vi "Get Configuration Version.vi"(8 "error in":errorcluster, 11 "data sharing framework custom device in":T1 format="%.0x") -> (0 "error out":errorcluster, 1 "version string":string, 2 "version":cluster{"major":u32, "minor":u32, "update":u32}, 3 "data sharing framework custom device out":T1 format="%.0x")   [LabVIEW 2020, in "Data Sharing Framework Custom Device Scripting.lvlib"]
doc: "Reads the version of the Data Sharing Framework custom device."
uses:
  Data Sharing Framework Custom Device Scripting.lvlib
  <vilib>/NI VeriStand/Custom Device API/Custom Device Item Ref.ctl
  DSF Shared.lvlib
  DSF System Explorer.lvlib
  <vilib>/NI VeriStand/Custom Device API/Custom Device API.lvlib
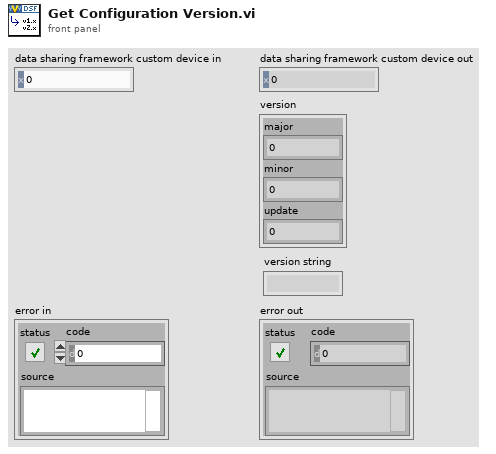
[diagram p1: front panel]
types:
  T1 = typedef "Custom Device API.lvlib/Custom Device Item Ref.ctl" = u64
  T2 = typedef "DSF Core.lvlibp/DSF Version Info.ctl" = cluster{"major":u32, "minor":u32, "fix":u32, "build":string}
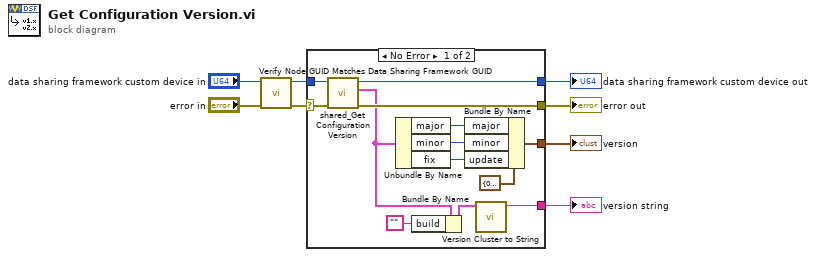
[diagram p0: block diagram]
diagram:
  n1 = call "Verify Node GUID Matches Data Sharing Framework GUID.vi"("error in"="error in", "data sharing framework custom device in"="data sharing framework custom device in") -> ("error out"=w1:errorcluster, "data sharing framework custom device out"=w2:T1)  [unwired: 8 in]
  n2 = case shown="No Error" w1 {
    selector: w1 -> [w16 w22]
    tunnel: [w21 w23] -> w8
    tunnel: [w20 w22] -> w7
    tunnel: [w9 _] -> w6
    tunnel: [w18 _] -> w5
    tunnel: w2 -> [w17 w23]
    frame No Error {
      n3 = call "shared_Get Configuration Version.vi"("error in (no error)"=w16, "Item Ref in"=w17) -> ("error out"=w20:errorcluster, "version"=w12:T2, "Item Ref out"=w21:T1)  [unwired: 7 in]
      n4 = Unbundle By Name(w12) -> ("major"=w13:u32, "minor"=w14:u32, "fix"=w15:u32)
      n5 = Bundle By Name(cluster=w12, "build"="") -> (w11:T2)
      n6 = Bundle By Name(cluster=cluster{"major":u32, "minor":u32, "update":u32} {"major"=0, "minor"=0, "update"=0} ("version"), "major"=w13, "minor"=w14, "update"=w15) -> (w18:cluster{"major":u32, "minor":u32, "update":u32})
      n7 = call "Version Cluster to String.vi"("version"=w11) -> ("version string"=w9:string)  [unwired: 9 in, 1 out]
    }
    frame Error {
    }
  }
  "data sharing framework custom device out" <- w8
  "error out" <- w7
  "version string" <- w6
  "version" <- w5
